vi "set up acquisition parameters.vi"() -> (1 "Kinetics":dbl format="%#_13g", 2 "Accumulation":dbl format="%#_13g", 3 "Exposure":dbl format="%#_13g")   [LabVIEW 2014]
uses:
  SubVIs/Initilize Globals.vi
  lib/Andorlib/atmcd32d.dll
  lib/Andorlib/atmcd32d.lvlib
panel:
  in  "EM CCD Gain":u16(slide)=230 scale=0.01..255.0
  in  "Acquisition Parameters":T1={"Readout Mode"=enum."Full Vertical Binning", "Set Acquisition Mode"=enum."(do nothing)", "Trigger Mode"=enum."Internal", "Exposure Time (s)"=0.0, "Accumulation Cycle (s)"=0.0, "Kinetic Cycle Time (s)"=0.0, "Number of Kinetics"=0, "Number of Accumulations"=0, "Set VS Speed"=0, "Pixel Rate"=enum."Standard CCD 3 Mhz 14 bits", "High Capacity?"=FALSE, "V Shift Amplitude"=enum."+1", "Preamp Gain"=enum."1.0"}
  in  "Shutter":i32(ring) items=["Auto", "Stay Open", "Always Closed"]
  out "error out":errorcluster
  in  "error in (no error)":errorcluster
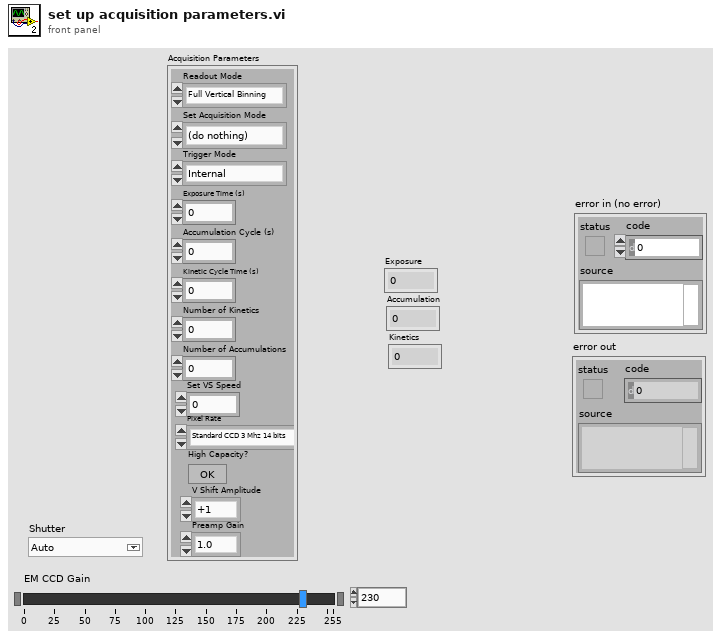
[diagram p1: front panel]
types:
  T1 = cluster{"Readout Mode":enum16{"Full Vertical Binning", "Multi-Track", "Random-Track", "Single-Track", "Image"}, "Set Acquisition Mode":enum16{"(do nothing)", "Single Scan", "Accumulate", "Kinetics", "Fast Kinetics", "Run till abort"}, "Trigger Mode":enum16{"Internal", "External"}, "Exposure Time (s)":dbl, "Accumulation Cycle (s)":dbl, "Kinetic Cycle Time (s)":dbl, "Number of Kinetics":i32, "Number of Accumulations":i32, "Set VS Speed":i32, "Pixel Rate":enum16{"EM CCD 10 Mhz 14 bits", "EM CCD 5 Mhz 14 bits", "EM CCD 3 Mhz 14 bits", "EM CCD 1 Mhz 16 bits", "Standard CCD 3 Mhz 14 bits", "Standard CCD 1 Mhz 16 bits"}, "High Capacity?":bool, "V Shift Amplitude":enum16{"normal", "+1", "+2", "+3", "+4"}, "Preamp Gain":enum16{"1.0", "2.4", "5.0"}}
  T2 = cluster{"Adc Channel":i32, "H Shift Setting":i32, "EM on?":bool}[]
  T3 = cluster{"H Bin":dbl, "V Bin":dbl, "Left":dbl, "Right":dbl, "Top":dbl, "Bottom":dbl}
  T4 = enum16{"Full Vertical Binning", "Multi-Track", "Random-Track", "Single-Track", "Image"}
  T5 = enum16{"(do nothing)", "Single Scan", "Accumulate", "Kinetics", "Fast Kinetics", "Run till abort"}
  T6 = enum16{"EM CCD 10 Mhz 14 bits", "EM CCD 5 Mhz 14 bits", "EM CCD 3 Mhz 14 bits", "EM CCD 1 Mhz 16 bits", "Standard CCD 3 Mhz 14 bits", "Standard CCD 1 Mhz 16 bits"}
  T7 = cluster{"Adc Channel":i32, "H Shift Setting":i32, "EM on?":bool}
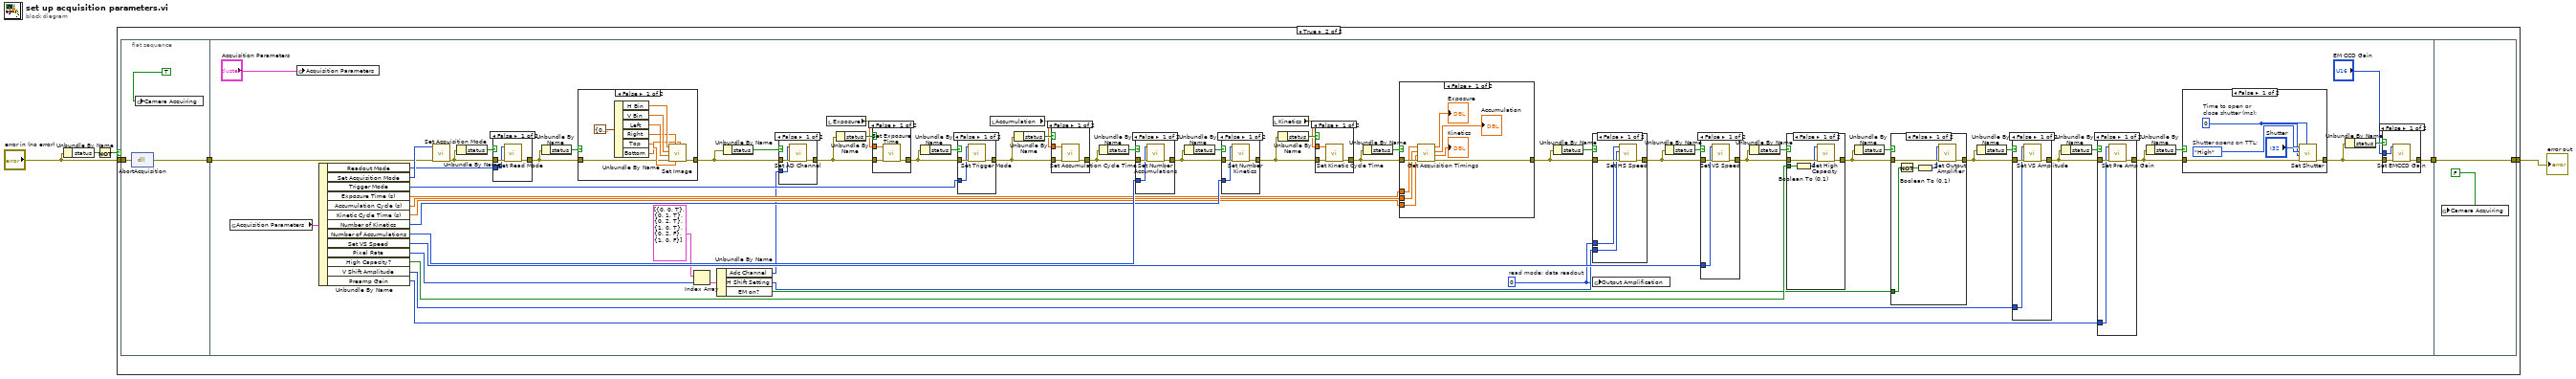
[diagram p0: block diagram]
diagram:
  n1 = Unbundle By Name("error in (no error)") -> ("status"=w4:bool)
  n2 = Not(x=w4) -> (.not. x?=w3:bool)
  n3 = case shown="True" w3 {
    tunnel: "error in (no error)" -> [w5 w8]
    tunnel: [w5 w7] -> w1
    frame False {
    }
    frame True {
      n4 = flat-sequence {
        tunnel: [w11] -> w9
        tunnel: w8 -> [w12]
        tunnel: w9 -> [w14]
        tunnel: [w13] -> w6
        tunnel: [w166] -> w7
        tunnel: w6 -> [w166]
        frame #0 {
          n5 = dll-call lib="C:/Users/Bakir/Desktop/LabFiles/Lambda2-Testing/lib/Andorlib/ATMCD32D.DLL" fn="AbortAcquisition" label="Call Library Function\nAbort"(error in=w12) -> (error out=w11:errorcluster)  [unwired: 2 in, 2 out]
          n6 = global write "Initilize Globals.vi" "Camera Acquiring"(TRUE) -> ()
        }
        frame #1 {
          w33 = 0  # read mode: data readout
          n7 = global read "Initilize Globals.vi" "Acquisition Parameters"() -> (w44:T1)
          n8 = global write "Initilize Globals.vi" "Acquisition Parameters"("Acquisition Parameters") -> ()
          n9 = Unbundle By Name(w44) -> ("Readout Mode"=w55:T4, "Set Acquisition Mode"=w56:T5, "Trigger Mode"=w54:enum16{"Internal", "External"}, "Exposure Time (s)"=w49:dbl, "Accumulation Cycle (s)"=w50:dbl, "Kinetic Cycle Time (s)"=w48:dbl, "Number of Kinetics"=w52:i32, "Number of Accumulations"=w53:i32, "Set VS Speed"=w51:i32, "Pixel Rate"=w40:T6, "High Capacity?"=w20:bool, "V Shift Amplitude"=w18:enum16{"normal", "+1", "+2", "+3", "+4"}, "Preamp Gain"=w17:enum16{"1.0", "2.4", "5.0"})
          n10 = call "Set Acquisition Mode.vi"("error in (no error)"=w14, "mode"=w56) -> ("error out"=w58:errorcluster)  [unwired: 8 in, 1 out]
          n11 = Unbundle By Name(w58) -> ("status"=w59:bool)
          n12 = case shown="False" w59 {
            tunnel: w58 -> [w121 w122]
            tunnel: [w120 w122] -> w42
            tunnel: w55 -> [w119 _]
            frame False {
              n13 = call "Set Read Mode.vi"("error in (no error)"=w121, "mode"=w119) -> ("error out"=w120:errorcluster)  [unwired: 8 in, 1 out]
            }
            frame True {
            }
          }
          n14 = Unbundle By Name(w42) -> ("status"=w43:bool)
          n15 = case shown="False" w43 {
            tunnel: w42 -> [w110 w118]
            tunnel: [w109 w118] -> w36
            frame False {
              n16 = Unbundle By Name(T3 {"H Bin"=0.0, "V Bin"=0.0, "Left"=0.0, "Right"=0.0, "Top"=0.0, "Bottom"=0.0} ("Image Size")) -> ("H Bin"=w116:dbl, "V Bin"=w115:dbl, "Left"=w114:dbl, "Right"=w113:dbl, "Top"=w112:dbl, "Bottom"=w111:dbl)
              n17 = call "Set Image.vi"("vend"=w111, "vstart"=w112, "hend"=w113, "error in (no error)"=w110, "hstart"=w114, "vbin"=w115, "hbin"=w116) -> ("error out"=w109:errorcluster)  [unwired: 3 in, 1 out]
            }
            frame True {
            }
          }
          n18 = Index Array(array=T2 [{"Adc Channel"=0, "H Shift Setting"=0, "EM on?"=TRUE}, {"Adc Channel"=0, "H Shift Setting"=1, "EM on?"=TRUE}, {"Adc Channel"=0, "H Shift Setting"=2, "EM on?"=TRUE}, {"Adc Channel"=1, "H Shift Setting"=0, "EM on?"=TRUE}, {"Adc Channel"=0, "H Shift Setting"=2, "EM on?"=FALSE}, {"Adc Channel"=1, "H Shift Setting"=0, "EM on?"=FALSE}], index=w40) -> (element=w39:T7)
          n19 = Unbundle By Name(w39) -> ("Adc Channel"=w35:i32, "H Shift Setting"=w34:i32, "EM on?"=w19:bool)
          n20 = Unbundle By Name(w36) -> ("status"=w38:bool)
          n21 = case shown="False" w38 {
            tunnel: [w106 w108] -> w37
            tunnel: w36 -> [w107 w108]
            tunnel: w35 -> [w105 _]
            frame False {
              n22 = call "Set AD Channel.vi"("error in (no error)"=w107, "channel"=w105) -> ("error out"=w106:errorcluster)  [unwired: 8 in, 1 out]
            }
            frame True {
            }
          }
          n23 = local read "Exposure"() -> (w47:dbl)
          n24 = Unbundle By Name(w37) -> ("status"=w57:bool)
          n25 = case shown="False" w57 {
            tunnel: w37 -> [w163 w164]
            tunnel: [w162 w164] -> w67
            tunnel: w47 -> [w161 _]
            frame False {
              n26 = call "Set Exposure Time.vi"("error in (no error)"=w163, "time"=w161) -> ("error out"=w162:errorcluster)  [unwired: 8 in, 1 out]
            }
            frame True {
            }
          }
          n27 = Unbundle By Name(w67) -> ("status"=w75:bool)
          n28 = case shown="False" w75 {
            tunnel: w67 -> [w159 w160]
            tunnel: [w158 w160] -> w66
            tunnel: w54 -> [w157 _]
            frame False {
              n29 = call "Set Trigger Mode.vi"("error in (no error)"=w159, "mode"=w157) -> ("error out"=w158:errorcluster)  [unwired: 8 in, 1 out]
            }
            frame True {
            }
          }
          n30 = local read "Accumulation"() -> (w46:dbl)
          n31 = Unbundle By Name(w66) -> ("status"=w74:bool)
          n32 = case shown="False" w74 {
            tunnel: w66 -> [w155 w156]
            tunnel: [w154 w156] -> w65
            tunnel: w46 -> [w153 _]
            frame False {
              n33 = call "Set Accumulation Cycle Time.vi"("error in (no error)"=w155, "time"=w153) -> ("error out"=w154:errorcluster)  [unwired: 8 in, 1 out]
            }
            frame True {
            }
          }
          n34 = Unbundle By Name(w65) -> ("status"=w73:bool)
          n35 = case shown="False" w73 {
            tunnel: w65 -> [w151 w152]
            tunnel: [w150 w152] -> w64
            tunnel: w53 -> [w149 _]
            frame False {
              n36 = call "Set Number Accumulations.vi"("error in (no error)"=w151, "number"=w149) -> ("error out"=w150:errorcluster)  [unwired: 8 in, 1 out]
            }
            frame True {
            }
          }
          n37 = Unbundle By Name(w64) -> ("status"=w72:bool)
          n38 = case shown="False" w72 {
            tunnel: w64 -> [w147 w148]
            tunnel: [w146 w148] -> w63
            tunnel: w52 -> [w145 _]
            frame False {
              n39 = call "Set Number Kinetics.vi"("error in (no error)"=w147, "number"=w145) -> ("error out"=w146:errorcluster)  [unwired: 8 in, 1 out]
            }
            frame True {
            }
          }
          n40 = local read "Kinetics"() -> (w45:dbl)
          n41 = Unbundle By Name(w63) -> ("status"=w71:bool)
          n42 = case shown="False" w71 {
            tunnel: w63 -> [w143 w144]
            tunnel: [w142 w144] -> w62
            tunnel: w45 -> [w141 _]
            frame False {
              n43 = call "Set Kinetic Cycle Time.vi"("error in (no error)"=w143, "time"=w141) -> ("error out"=w142:errorcluster)  [unwired: 8 in, 1 out]
            }
            frame True {
            }
          }
          n44 = Unbundle By Name(w62) -> ("status"=w70:bool)
          n45 = case shown="False" w70 {
            tunnel: w62 -> [w139 w140]
            tunnel: [w138 w140] -> w61
            tunnel: w50 -> [w137 _]
            tunnel: w49 -> [w136 _]
            tunnel: w48 -> [w135 _]
            frame False {
              n46 = call "Get Acquisition Timings.vi"("error in (no error)"=w139, "kinetic"=w135, "accumulate"=w137, "exposure"=w136) -> ("error out"=w138:errorcluster, "kinetic out"=→"Kinetics":sgl, "accumulate out"=→"Accumulation":sgl, "exposure out"=→"Exposure":sgl)  [unwired: 3 in, 1 out]
            }
            frame True {
            }
          }
          n47 = Unbundle By Name(w61) -> ("status"=w69:bool)
          n48 = case shown="False" w69 {
            tunnel: w61 -> [w130 w131]
            tunnel: [w129 w131] -> w60
            tunnel: w34 -> [w128 _]
            tunnel: w33 -> [w127 _]
            frame False {
              n49 = call "Set HS Speed.vi"("error in (no error)"=w130, "index"=w128, "typ"=w127) -> ("error out"=w129:errorcluster)  [unwired: 7 in, 1 out]
            }
            frame True {
            }
          }
          n50 = global write "Initilize Globals.vi" "Output Amplification"(w33) -> ()
          n51 = Unbundle By Name(w60) -> ("status"=w68:bool)
          n52 = case shown="False" w68 {
            tunnel: w60 -> [w125 w126]
            tunnel: [w124 w126] -> w26
            tunnel: w51 -> [w123 _]
            frame False {
              n53 = call "Set VS Speed.vi"("error in (no error)"=w125, "index"=w123) -> ("error out"=w124:errorcluster)  [unwired: 8 in, 1 out]
            }
            frame True {
            }
          }
          n54 = Unbundle By Name(w26) -> ("status"=w32:bool)
          n55 = case shown="False" w32 {
            tunnel: [w102 w104] -> w25
            tunnel: w26 -> [w103 w104]
            tunnel: w20 -> [w100 _]
            frame False {
              n56 = Boolean To (0,1)(Boolean=w100) -> (0, 1=w101:i16)
              n57 = call "Set High Capacity.vi"("error in (no error)"=w103, "state"=w101) -> ("error out"=w102:errorcluster)  [unwired: 8 in, 1 out]
            }
            frame True {
            }
          }
          n58 = Unbundle By Name(w25) -> ("status"=w31:bool)
          n59 = case shown="False" w31 {
            tunnel: [w97 w99] -> w24
            tunnel: w25 -> [w98 w99]
            tunnel: w19 -> [w94 _]
            frame False {
              n60 = Not(x=w94) -> (.not. x?=w95:bool)
              n61 = Boolean To (0,1)(Boolean=w95) -> (0, 1=w96:i16)
              n62 = call "Set Output Amplifier.vi"("error in (no error)"=w98, "typ"=w96) -> ("error out"=w97:errorcluster)  [unwired: 8 in, 1 out]
            }
            frame True {
            }
          }
          n63 = Unbundle By Name(w24) -> ("status"=w30:bool)
          n64 = case shown="False" w30 {
            tunnel: [w91 w93] -> w23
            tunnel: w24 -> [w92 w93]
            tunnel: w18 -> [w90 _]
            frame False {
              n65 = call "Set VS Amplitude.vi"("error in (no error)"=w92, "index"=w90) -> ("error out"=w91:errorcluster)  [unwired: 8 in, 1 out]
            }
            frame True {
            }
          }
          n66 = Unbundle By Name(w23) -> ("status"=w29:bool)
          n67 = case shown="False" w29 {
            tunnel: [w87 w89] -> w22
            tunnel: w23 -> [w88 w89]
            tunnel: w17 -> [w86 _]
            frame False {
              n68 = call "Set Pre Amp Gain.vi"("error in (no error)"=w88, "index"=w86) -> ("error out"=w87:errorcluster)  [unwired: 8 in, 1 out]
            }
            frame True {
            }
          }
          n69 = Unbundle By Name(w22) -> ("status"=w28:bool)
          n70 = case shown="False" w28 {
            tunnel: [w83 w85] -> w21
            tunnel: w22 -> [w84 w85]
            frame False {
              w80 = 0  # Time to open or close shutter (ms):
              w82 = enum16{"Low", "High"}."High"  # Shutter opens on TTL:
              n71 = call "Set Shutter.vi"("openingtime"=w80, "error in (no error)"=w84, "closingtime"=w80, "mode"="Shutter", "typ"=w82) -> ("error out"=w83:errorcluster)  [unwired: 5 in, 1 out]
            }
            frame True {
            }
          }
          n72 = Unbundle By Name(w21) -> ("status"=w27:bool)
          n73 = case shown="False" w27 {
            tunnel: [w77 w79] -> w13
            tunnel: w21 -> [w78 w79]
            tunnel: "EM CCD Gain" -> [w76 _]
            frame False {
              n74 = call "Set EMCCD Gain.vi"("error in (no error)"=w78, "gain"=w76) -> ("error out"=w77:errorcluster)  [unwired: 8 in, 1 out]
            }
            frame True {
            }
          }
        }
        frame #2 {
          n75 = global write "Initilize Globals.vi" "Camera Acquiring"(FALSE) -> ()
        }
      }
    }
  }
  "error out" <- w1
